vi "Post-Install Custom Action - Generator.vi"() -> (0 "error out":errorcluster)   [LabVIEW 2021]
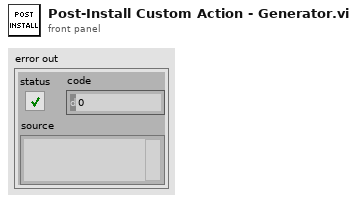
[diagram p1: front panel]
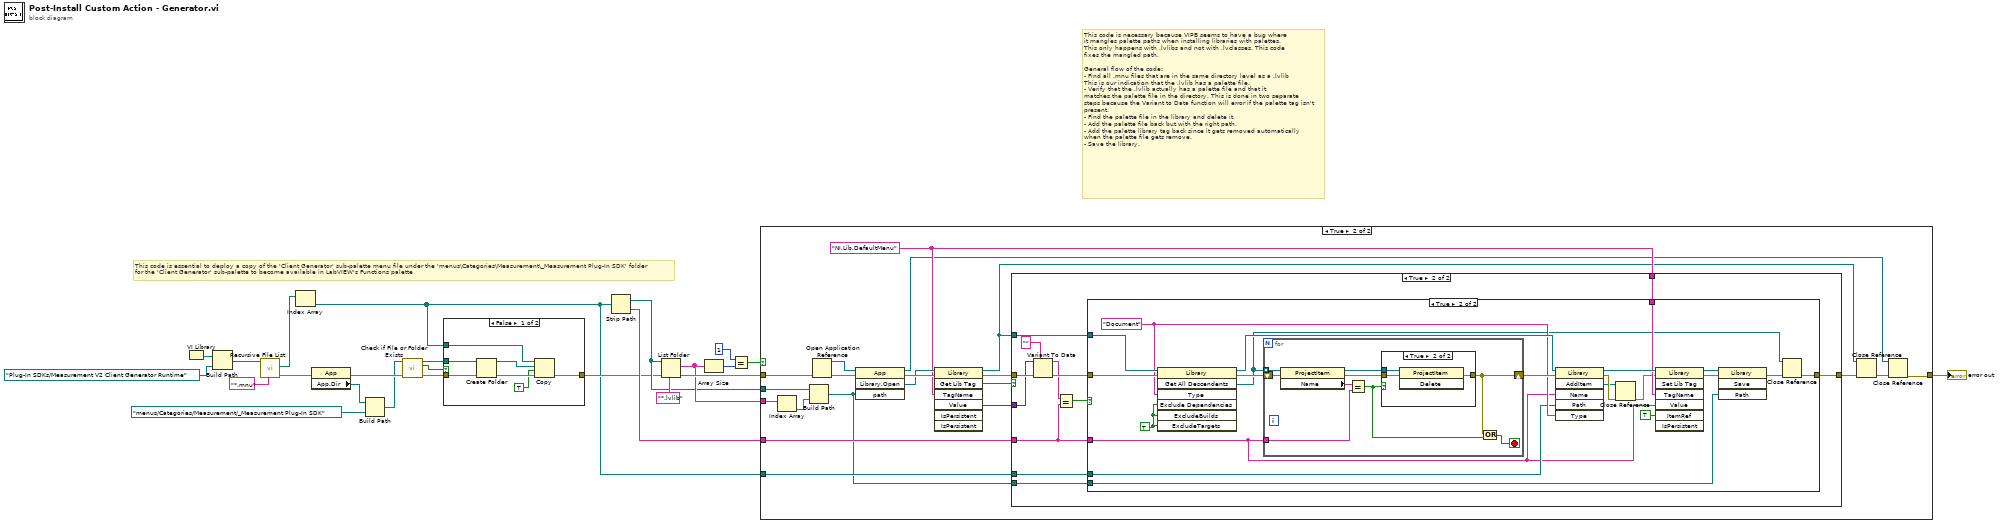
[diagram p0: block diagram]
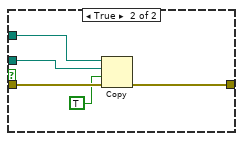
[diagram p2: hidden frame]
diagram:
  # "This code is essential to deploy a copy of the 'Client Generator' sub-palette menu file under the 'menus\\Categories\\Measurement\\_Measurement Plug-In SDK' folder\nfor the 'Client Generator' sub-palette to become available in LabVIEW's Functions palette"
  # "This code is necessary because VIPB seems to have a bug where\nit mangles palette paths when installing libraries with palettes.\nThis only happens with .lvlibs and not with .lvclasses. This code\nfixes the mangled path.\n\nGeneral flow of the code:\n- Find all .mnu files that are in the same directory level as a .lvlib\nThis is our indication that the .lvlib has a palette file.\n- Verify that the .lvlib actually has a palette file and that it\nmatches the palette file in the directory. This is done in two separate\nsteps because the Variant to Data function will error if the palette tag isn't\npresent.\n- Find the palette file in the library and delete it.\n- Add the palette file back but with the right path.\n- Add the palette library tag back since it gets removed automatically\nwhen the palette file gets remove.\n- Save the library."
  n1 = VI Library() -> (path=w2:path)
  n2 = Build Path(base path=w2, name or relative path=path "Plug-In SDKs/Measurement V2 Client Generator Runtime") -> (appended path=w24:path)
  n3 = call <vilib>:"Recursive File List.vi"("pattern"="*.mnu", "Folder Path"=w24) -> ("error out"=w22:errorcluster, "All Files in Dir"=w11:path[])  [unwired: 5 in, 3 out]
  n4 = Index Array(array=w11) -> (element=w1:path)  [unwired: 1 in]
  n5 = property class="App"(error in=w22) -> (error out=w10:errorcluster, "App.Dir"=w9:path)  [unwired: 1 in, 1 out]
  n6 = Build Path(base path=w9, name or relative path=path "menus/Categories/Measurement/_Measurement Plug-In SDK") -> (appended path=w7:path)
  n7 = call <vilib>:"Check if File or Folder Exists.vi"("error in (no error)"=w10, "path"=w7) -> ("error out"=w8:errorcluster, "file or folder exists?"=w6:bool, "dup path"=w5:path)  [unwired: 7 in]
  n8 = case shown="False" w6 {
    tunnel: [w28 w36] -> w12
    tunnel: w8 -> [w31 w35]
    tunnel: w5 -> [w29 w34]
    tunnel: w1 -> [w27 w33]
    frame False {
      n9 = Create Folder(path (use dialog)=w29, error in=w31) -> (created path=w26:path, error out=w30:errorcluster)  [unwired: 1 in, 1 out]
      n10 = Copy(8:w30, 9:TRUE ("overwrite (F)"), 10:w26, 11:w27) -> (0:w28:errorcluster)  [unwired: 1 in, 2 out]
    }
    frame True {
      n11 = Copy(8:w35, 9:TRUE ("overwrite (F)"), 10:w34, 11:w33) -> (0:w36:errorcluster)  [unwired: 1 in, 2 out]
    }
  }
  n12 = Strip Path(path=w1) -> (stripped path=w13:path, name=w17:string)
  n13 = List Folder(path=w13, pattern="*.lvlib", error in=w12) -> (filenames=w14:string[], error out=w16:errorcluster)  [unwired: 1 in, 2 out]
  n14 = Array Size(array=w14) -> (size(s)=w20:i32)
  n15 = Equal?(x=1, y=w20) -> (x = y?=w18:bool)
  n16 = case shown="True" w18 {
    tunnel: w16 -> [w37 w54]
    tunnel: w14 -> [_ w57]
    tunnel: [w37 w42] -> w21
    tunnel: w17 -> [_ w47]
    tunnel: w1 -> [_ w46]
    tunnel: w13 -> [_ w40]
    frame False {
    }
    frame True {
      w49 = "NI.Lib.DefaultMenu" ("Tag Name")
      n17 = Index Array(array=w57) -> (element=w39:string)  [unwired: 1 in]
      n18 = Build Path(base path=w40, name or relative path=w39) -> (appended path=w38:path)
      n19 = Open Application Reference(8:w54) -> (0:w56:errorcluster, 3:w55:refnum<vi>)  [unwired: 3 in]
      n20 = invoke class="App" method="Library.Open"(reference=w55, error in=w56, "path"=w38) -> (reference out=w41:refnum<vi>, error out=w53:errorcluster, "Open Library"=w50:refnum<vi>)  [unwired: 1 in, 1 out]
      n21 = invoke class="Library" method="Get Lib Tag"(reference=w50, error in=w53, "TagName"=w49) -> (reference out=w44:refnum<vi>, error out=w51:errorcluster, "GetTag"=w48:bool, "Value"=w52:variant)  [unwired: 4 in, 3 out]
      n22 = case shown="True" w48 {
        tunnel: w52 -> [_ w65]
        tunnel: w51 -> [w58 w66]
        tunnel: [w58 w70] -> w45
        tunnel: w44 -> [_ w69]
        tunnel: w49 -> [_ w68]
        tunnel: w38 -> [_ w67]
        tunnel: w47 -> [_ w60]
        tunnel: w46 -> [_ w59]
        frame False {
        }
        frame True {
          n23 = Variant To Data(error in=w66, type="", Variant=w65) -> (data=w62:string, error out=w64:errorcluster)
          n24 = Equal?(x=w62, y=w60) -> (x = y?=w61:bool)
          n25 = case shown="True" w61 {
            tunnel: [w71 w72] -> w70
            tunnel: w69 -> [_ w92]
            tunnel: w68 -> [_ w85]
            tunnel: w67 -> [_ w83]
            tunnel: w64 -> [w71 w82]
            tunnel: w60 -> [_ w78]
            tunnel: w59 -> [_ w79]
            frame False {
            }
            frame True {
              w80 = "Document" ("Type")
              w91 = TRUE ("ExcludeDependencies")
              n26 = invoke class="Library" method="Get All Descendents"(reference=w92, error in=w82, "Type"=w80, "Exclude Dependencies"=w91, "ExcludeBuilds"=w91, "ExcludeTargets"=w91) -> (reference out=w81:refnum<vi>, error out=w90:errorcluster, "All Descendents"=w76:refnum<vi>[])  [unwired: 1 in, 4 out]
              n27 = for {
                tunnel: w76 -> [w101] mode=indexing
                shift-right: [w94] -> w89
                shift-left: w90 -> [w97]
                tunnel: w78 -> [w96]
                stop <- w95 stop-if-true
                n28 = property class="ProjectItem"(reference=w101, error in=w97) -> (reference out=w99:refnum<vi>, error out=w98:errorcluster, "Name"=w100:string)
                n29 = Equal?(x=w100, y=w96) -> (x = y?=w93:bool)
                n30 = case shown="True" w93 {
                  tunnel: w99 -> [_ w105]
                  tunnel: w98 -> [w102 w103]
                  tunnel: [w102 w104] -> w94
                  frame False {
                  }
                  frame True {
                    n31 = invoke class="ProjectItem" method="Delete"(reference=w105, error in=w103) -> (error out=w104:errorcluster)  [unwired: 1 in, 2 out]
                  }
                }
                n32 = Or(x=w94, y=w93) -> (x .or. y?=w95:bool)
              }
              n33 = invoke class="Library" method="AddItem"(reference=w81, error in=w89, "Name"=w78, "Path"=w79, "Type"=w80) -> (reference out=w88:refnum<vi>, error out=w75:errorcluster, "AddItem"=w74:refnum<vi>)  [unwired: 1 in, 3 out]
              n34 = Close Reference(reference=w74, error in (no error)=w75) -> (error out=w73:errorcluster)
              n35 = invoke class="Library" method="Set Lib Tag"(reference=w88, error in=w73, "TagName"=w85, "Value"=w78, "ItemRef"=TRUE ("Is Persistent")) -> (reference out=w87:refnum<vi>, error out=w86:errorcluster)  [unwired: 2 in, 5 out]
              n36 = invoke class="Library" method="Save"(reference=w87, error in=w86, "Path"=w83) -> (error out=w77:errorcluster)  [unwired: 1 in, 3 out]
              n37 = Close Reference(reference=w76, error in (no error)=w77) -> (error out=w72:errorcluster)
            }
          }
        }
      }
      n38 = Close Reference(reference=w44, error in (no error)=w45) -> (error out=w43:errorcluster)
      n39 = Close Reference(reference=w41, error in (no error)=w43) -> (error out=w42:errorcluster)
    }
  }
  "error out" <- w21
